vi "set_encoding.vi"(8 "error in (no error)":errorcluster, 11 "Process StartInfo Ref in":refnum<k24>) -> (0 "error out":errorcluster, 3 "Process StartInfo Ref out":refnum<k24>)   [LabVIEW 2015, in "dotnet_system_exec.lvclass"]
doc: "Set StdOut and StdErr encoding to OEM Code Page."
uses:
  dotnet_system_exec.lvclass
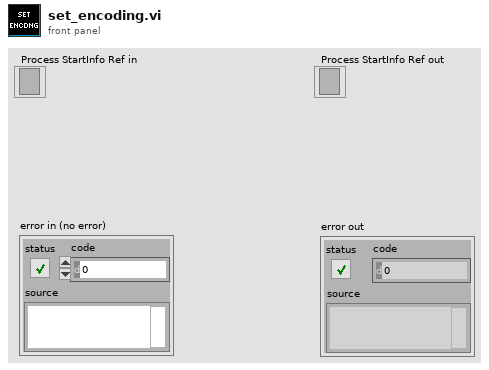
[diagram p1: front panel]
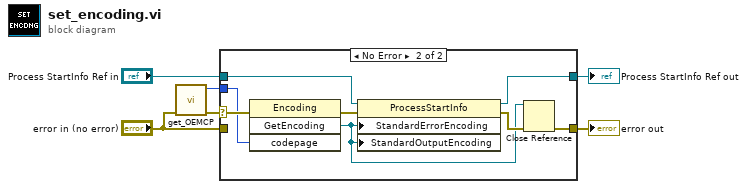
[diagram p0: block diagram]
diagram:
  n1 = call "get_OEMCP.vi"("error in (no error)"="error in (no error)") -> ("error out"=w2:errorcluster, "OEMCodePage"=w1:i32)  [unwired: 9 in]
  n2 = case shown="No Error" w2 {
    selector: w2 -> [_ w16]
    tunnel: "Process StartInfo Ref in" -> [w8 w15]
    tunnel: [w8 w14] -> w5
    tunnel: [w7 w10] -> w4
    tunnel: w1 -> [_ w13]
    tunnel: "error in (no error)" -> [w7 _]
    frame Error {
    }
    frame No Error {
      n3 = invoke class="Encoding" method="GetEncoding"(error in=w16, "codepage"=w13) -> (error out=w12:errorcluster, "GetEncoding"=w9:refnum<k24>)  [unwired: 2 in, 2 out]
      n4 = property class="ProcessStartInfo"(reference=w15, error in=w12, "StandardErrorEncoding"=w9, "StandardOutputEncoding"=w9) -> (reference out=w14:refnum<k24>, error out=w11:errorcluster)
      n5 = Close Reference(reference=w9, error in (no error)=w11) -> (error out=w10:errorcluster)
    }
  }
  "Process StartInfo Ref out" <- w5
  "error out" <- w4
